vi "Wire All Terminals_core.vi"(8 "error in (no error)":errorcluster, 9 "User string":string, 10 "Create constants?":bool, 11 "SelList[]":refnum<vi>[](array[refnum])) -> (0 "error out":errorcluster, 3 "changes made?":bool)   [LabVIEW 2017]
doc: "Creates controls and indicators for all unwired inputs and outputs of the selected block diagram object(s). If 'shift' is also pressed, creates constants for all unwired inputs of the selected block diagram object(s).\n\nDefault Shortcut - [D]"
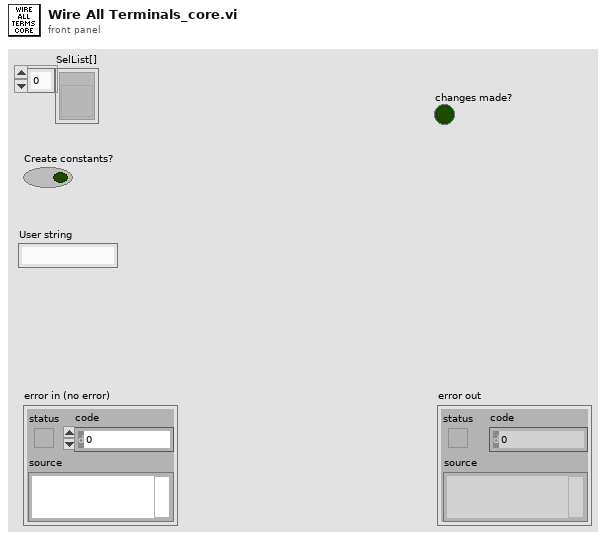
[diagram p1: front panel]
types:
  T1 = enum16{"Invalid Wire Rule", "Required", "Recommended", "Optional", "Dynamic Dispatch"}[]
  T2 = typedef "VariantType.lvlib/Type.ctl" = enum8{"Invalid Type", "Void", "I8", "I16", "I32", "I64", "U8", "U16", "U32", "U64", "Single Float", "Double Float", "Extended Float", "Single Complex", "Double Complex", "Extended Complex", "Enum U8", "Enum U16", "Enum U32", "Enum U64", "Single Float With Unit", "Double Float With Unit", "Extended Float With Unit", "Single Complex with Unit", "Double Complex with Unit", "Extended Complex with Unit", "Boolean", "String", "Path", "Picture", "Tag", "Array", "Cluster", "Variant", "LV Variant", "Waveform", "Timestamp", "Digital Waveform", "Digital Data", "ExpressData", "Refnum", "External Data", "VI", "Poly VI", "LabVIEW Class Instance", "Fixed Point"}
  T3 = enum16{"Invalid Wire Rule", "Required", "Recommended", "Optional"}
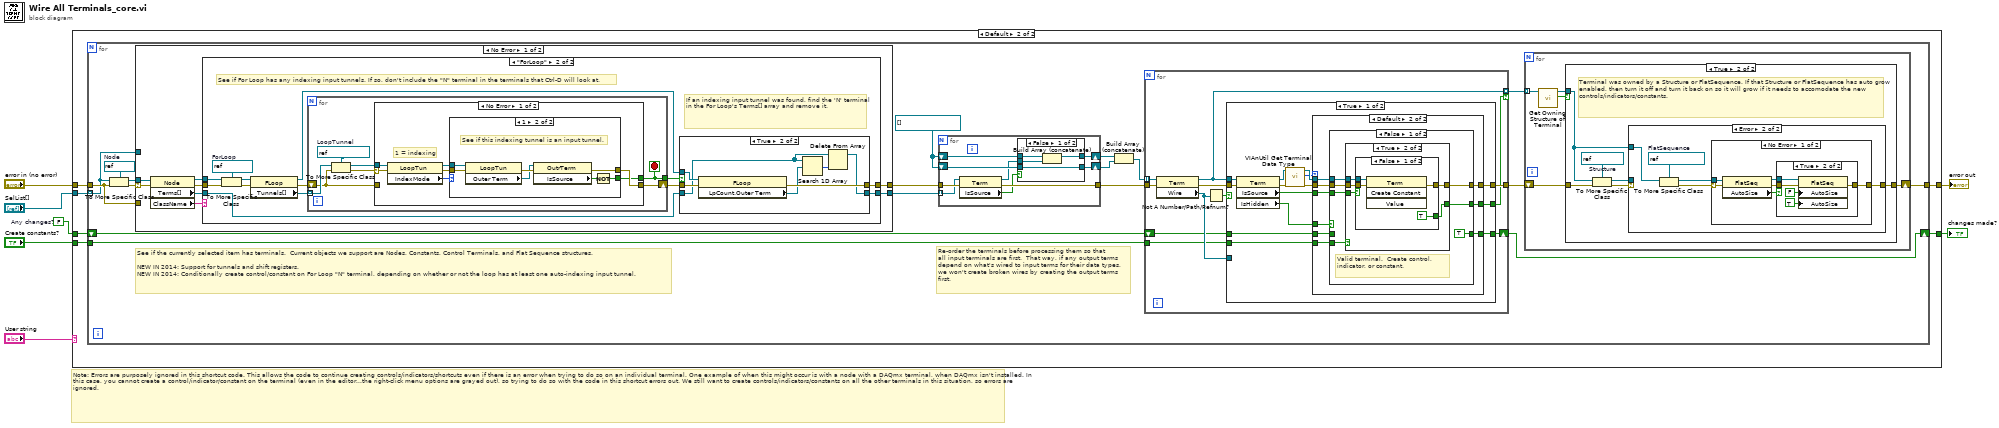
[diagram p0: block diagram]
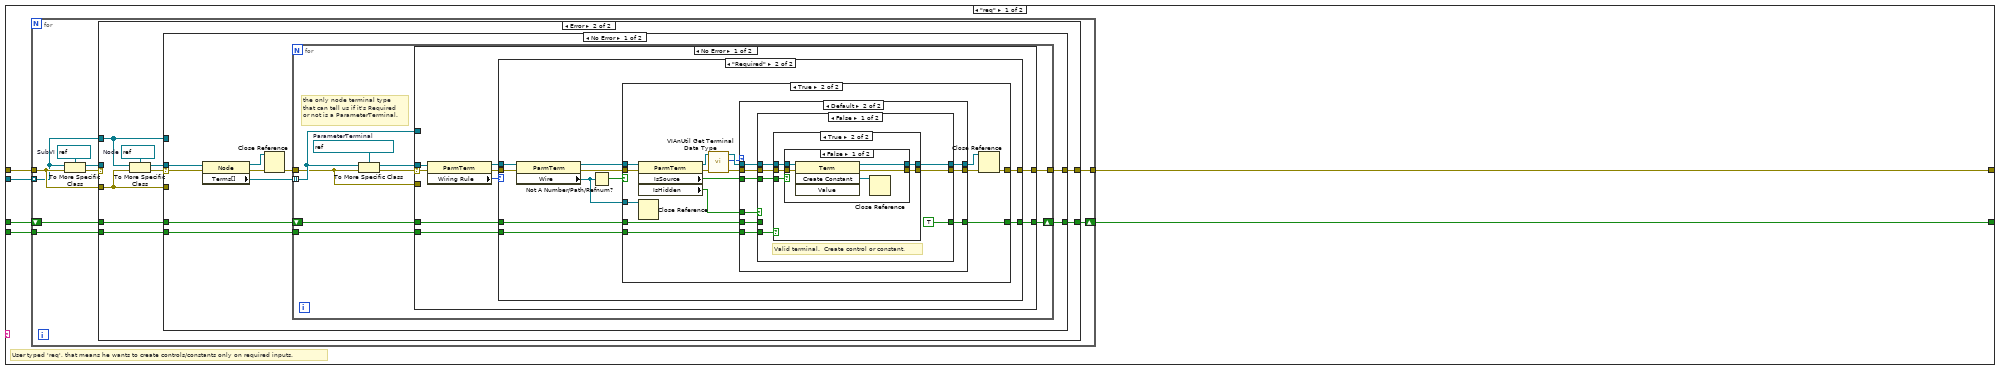
[diagram p2: hidden frame]
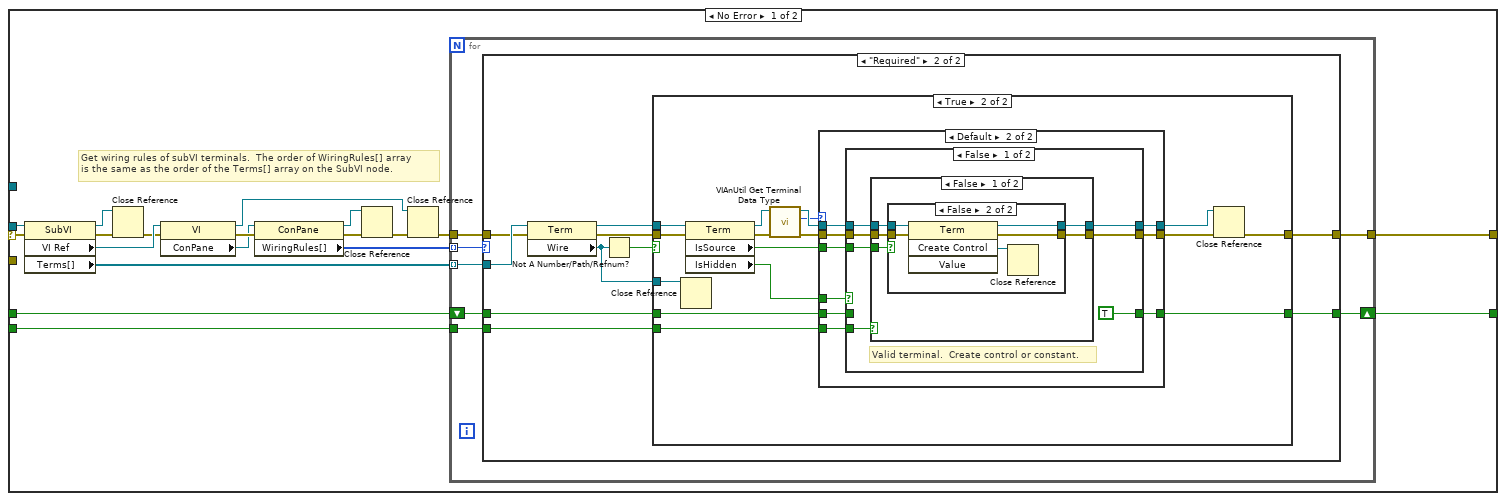
[diagram p3: hidden frame]
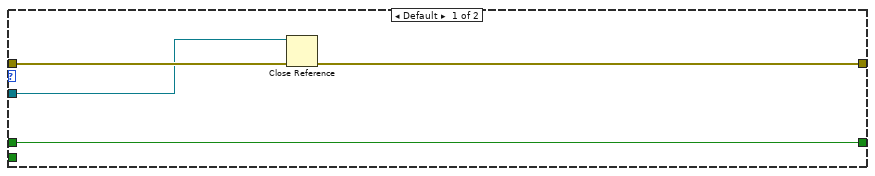
[diagram p4: hidden frame]
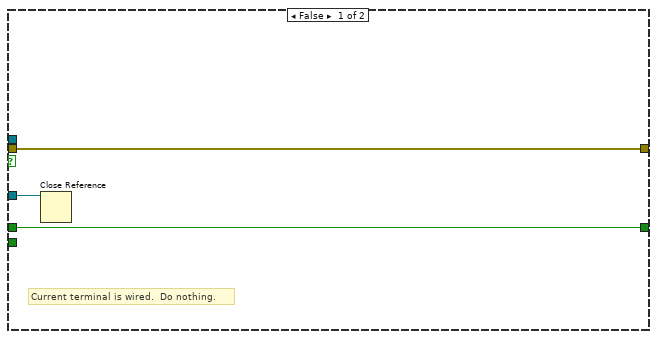
[diagram p5: hidden frame]
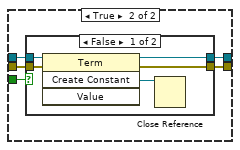
[diagram p8: hidden frame]
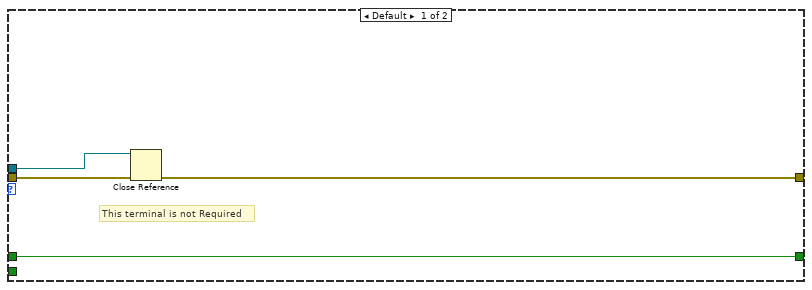
[diagram p11: hidden frame]
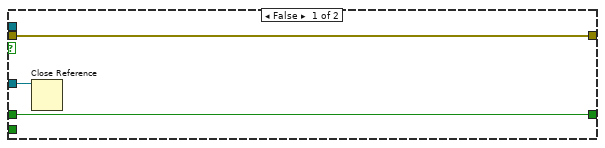
[diagram p12: hidden frame]
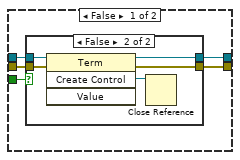
[diagram p14: hidden frame]
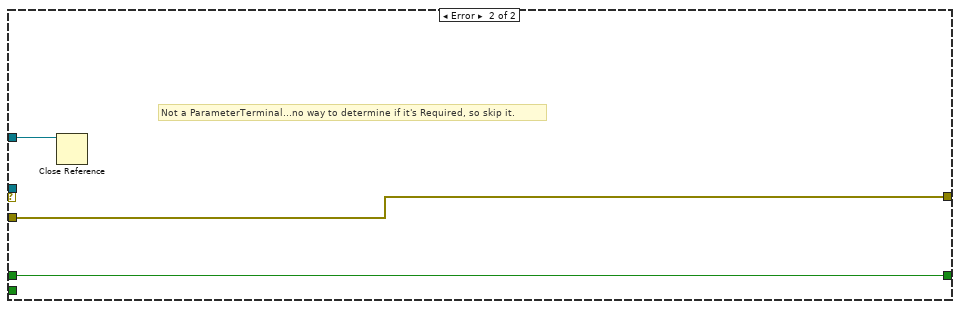
[diagram p18: hidden frame]
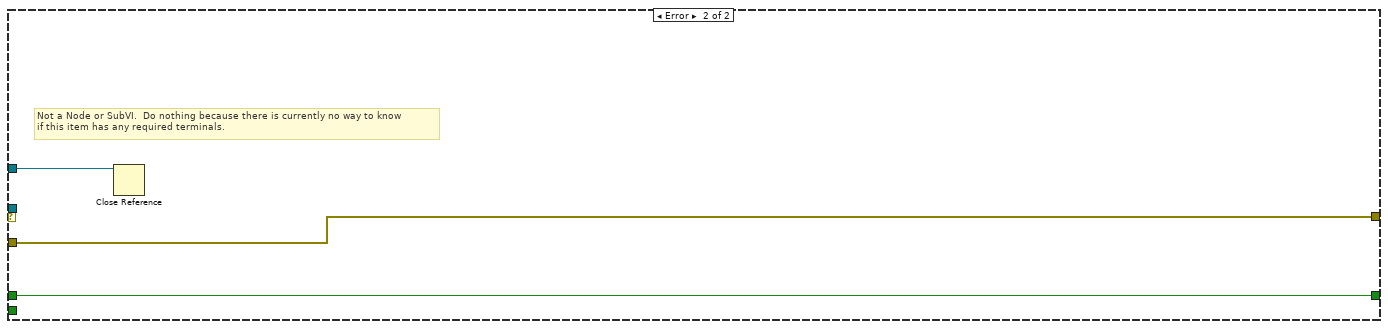
[diagram p19: hidden frame]
diagram:
  w7 = FALSE  # Any changes?
  # "Note: Errors are purposely ignored in this shortcut code. This allows the code to continue creating controls/indicators/shortcuts even if there is an error when trying to do so on an individual terminal. One example of when this might occur is with a node with a DAQmx terminal, when DAQmx isn't installed. In this case, you cannot create a control/indicator/constant on the terminal (even in the editor...the right-click menu options are grayed out), so trying to do so with the code in this shortcut errors out. We still want to create controls/indicators/constants on all the other terminals in this situation, so errors are ignored."
  n1 = case shown="Default" "User string" {
    tunnel: "Create constants?" -> [w8 w255]
    tunnel: w7 -> [w13 w254]
    tunnel: [w12 w253] -> w4
    tunnel: [w9 w252] -> w5
    tunnel: "SelList[]" -> [w11 w251]
    tunnel: "error in (no error)" -> [w10 w250]
    frame "req" {
      # "User typed 'req', that means he wants to create controls/constants only on required inputs."
      n2 = for {
        shift-right: [w17] -> w12
        shift-left: w13 -> [w19]
        tunnel: w11 -> [w14] mode=indexing
        tunnel: w8 -> [w16]
        tunnel: w10 -> [w15]
        tunnel: [w18] -> w9
        w22 = refnum<vi> refnum  # SubVI
        n3 = To More Specific Class(target class=w22, reference=w14, error in=w15) -> (specific class reference=w20:refnum<vi>, error out=w21:errorcluster)
        n4 = case shown="Error" w21 {
          selector: w21 -> [w40 _]
          tunnel: w20 -> [w41 _]
          tunnel: w19 -> [w27 w129]
          tunnel: [w30 w131] -> w18
          tunnel: [w26 w130] -> w17
          tunnel: w16 -> [w25 w128]
          tunnel: w15 -> [_ w134]
          tunnel: w14 -> [_ w132]
          frame No Error {
            # "Get wiring rules of subVI terminals.  The order of WiringRules[] array\nis the same as the order of the Terms[] array on the SubVI node."
            n5 = property class="SubVI"(reference=w41, error in=w40) -> (reference out=w23:refnum<vi>, error out=w39:errorcluster, "VI Ref"=w38:refnum<vi>, "Terms[]"=w28:refnum<vi>[])
            n6 = Close Reference(reference=w23, error in (no error)=w39) -> (error out=w24:errorcluster)
            n7 = property class="VI"(reference=w38, error in=w24) -> (reference out=w32:refnum<vi>, error out=w37:errorcluster, "ConPane"=w36:refnum<vi>)
            n8 = property class="ConPane"(reference=w36, error in=w37) -> (reference out=w34:refnum<vi>, error out=w35:errorcluster, "WiringRules[]"=w29:T1)
            n9 = Close Reference(reference=w34, error in (no error)=w35) -> (error out=w33:errorcluster)
            n10 = Close Reference(reference=w32, error in (no error)=w33) -> (error out=w31:errorcluster)
            n11 = for {
              tunnel: w29 -> [w47] mode=indexing
              tunnel: w28 -> [w46] mode=indexing
              shift-right: [w43] -> w26
              shift-left: w27 -> [w44]
              tunnel: w25 -> [w42]
              tunnel: w31 -> [w48]
              tunnel: [w45] -> w30
              n12 = case shown="\"Required\"" w47 {
                tunnel: w48 -> [w52 w54]
                tunnel: w46 -> [w49 w58]
                tunnel: [w51 w59] -> w45
                tunnel: w44 -> [w50 w62]
                tunnel: [w50 w60] -> w43
                tunnel: w42 -> [_ w61]
                frame Default {
                  n13 = Close Reference(reference=w49, error in (no error)=w52) -> (error out=w51:errorcluster)
                }
                frame "Required" {
                  n14 = property class="Term"(reference=w58, error in=w54) -> (reference out=w57:refnum<vi>, error out=w53:errorcluster, "Wire"=w55:refnum<vi>)
                  n15 = Not A Number/Path/Refnum?(number/path/refnum=w55) -> (NaN/Path/Refnum?=w56:bool)
                  n16 = case shown="True" w56 {
                    tunnel: w62 -> [w63 w77]
                    tunnel: w61 -> [_ w76]
                    tunnel: [w63 w75] -> w60
                    tunnel: [w64 w74] -> w59
                    tunnel: w53 -> [w64 w73]
                    tunnel: w57 -> [_ w67]
                    tunnel: w55 -> [w65 w66]
                    frame False {
                      # "Current terminal is wired.  Do nothing."
                      n17 = Close Reference(reference=w65) -> ()  [unwired: 1 in, 1 out]
                    }
                    frame True {
                      n18 = Close Reference(reference=w66) -> ()  [unwired: 1 in, 1 out]
                      n19 = property class="Term"(reference=w67, error in=w73) -> (reference out=w70:refnum<vi>, error out=w72:errorcluster, "IsSource"=w81:bool, "IsHidden"=w78:bool)
                      n20 = call <vilib>:"VIAnUtil Get Terminal Data Type.vi"("error in (no error)"=w72, "Terminal"=w70) -> ("error out"=w71:errorcluster, "Data Type"=w68:T2, "dup  Terminal"=w69:refnum<vi>)  [unwired: 6 in, 1 out]
                      n21 = case shown="Default" w68 {
                        tunnel: [w84 w93] -> w75
                        tunnel: w81 -> [_ w92]
                        tunnel: w69 -> [w82 w91]
                        tunnel: [w83 w90] -> w80
                        tunnel: [w82 w89] -> w79
                        tunnel: w71 -> [w83 w88]
                        tunnel: w77 -> [w84 w85]
                        tunnel: w76 -> [_ w87]
                        tunnel: w78 -> [_ w86]
                        frame "Invalid Type", "Void" {
                          # "Current terminal is void (like an empty terminal on\na subVI).  Do nothing."
                        }
                        frame Default {
                          n22 = case shown="False" w86 {
                            tunnel: [TRUE w125] -> w93
                            tunnel: w92 -> [w99 _]
                            tunnel: w91 -> [w98 w126]
                            tunnel: [w97 w127] -> w90
                            tunnel: [w96 w126] -> w89
                            tunnel: w88 -> [w95 w127]
                            tunnel: w87 -> [w94 _]
                            tunnel: w85 -> [_ w125]
                            frame False {
                              # "Valid terminal.  Create control or constant."
                              n23 = case shown="False" w94 {
                                tunnel: w99 -> [w105 w117]
                                tunnel: w98 -> [w104 w116]
                                tunnel: [w103 w115] -> w97
                                tunnel: [w102 w114] -> w96
                                tunnel: w95 -> [w101 w113]
                                frame False {
                                n24 = case shown="False" w105 {
                                tunnel: w101 -> [w106 w112]
                                tunnel: w104 -> [w107 w110]
                                tunnel: [w106 w111] -> w103
                                tunnel: [w107 w109] -> w102
                                frame True {
                                }
                                frame False {
                                n25 = invoke class="Term" method="Create Control"(reference=w110, error in=w112) -> (reference out=w109:refnum<vi>, error out=w111:errorcluster, "Create Control"=w108:refnum<vi>)  [unwired: 2 in, 1 out]
                                n26 = Close Reference(reference=w108) -> ()  [unwired: 1 in, 1 out]
                                }
                                }
                                }
                                frame True {
                                n27 = case shown="False" w117 {
                                tunnel: w113 -> [w122 w124]
                                tunnel: w116 -> [w120 w123]
                                tunnel: [w121 w124] -> w115
                                tunnel: [w119 w123] -> w114
                                frame False {
                                n28 = invoke class="Term" method="Create Constant"(reference=w120, error in=w122) -> (reference out=w119:refnum<vi>, error out=w121:errorcluster, "Create Constant"=w118:refnum<vi>)  [unwired: 2 in, 1 out]
                                n29 = Close Reference(reference=w118) -> ()  [unwired: 1 in, 1 out]
                                }
                                frame True {
                                }
                                }
                                }
                              }
                            }
                            frame True {
                              # "Do not attempt to create inputs/outputs\non hidden terminals (like Dynamic Event terms\non an Event Structure that aren't showing)"
                            }
                          }
                        }
                      }
                      n30 = Close Reference(reference=w79, error in (no error)=w80) -> (error out=w74:errorcluster)
                    }
                  }
                }
              }
            }
          }
          frame Error {
            w136 = refnum<vi> refnum  # Node
            n31 = To More Specific Class(target class=w136, reference=w132, error in=w134) -> (specific class reference=w133:refnum<vi>, error out=w135:errorcluster)
            n32 = case shown="No Error" w135 {
              selector: w135 -> [w146 _]
              tunnel: w134 -> [_ w248]
              tunnel: w133 -> [w145 _]
              tunnel: w132 -> [_ w249]
              tunnel: [w138 w248] -> w131
              tunnel: [w139 w247] -> w130
              tunnel: w129 -> [w140 w247]
              tunnel: w128 -> [w137 _]
              frame No Error {
                n33 = property class="Node"(reference=w145, error in=w146) -> (reference out=w143:refnum<vi>, error out=w144:errorcluster, "Terms[]"=w141:refnum<vi>[])
                n34 = Close Reference(reference=w143, error in (no error)=w144) -> (error out=w142:errorcluster)
                n35 = for {
                  tunnel: w141 -> [w150] mode=indexing
                  shift-right: [w151] -> w139
                  shift-left: w140 -> [w152]
                  tunnel: w137 -> [w147]
                  tunnel: w142 -> [w149]
                  tunnel: [w148] -> w138
                  w155 = refnum<vi> refnum  # ParameterTerminal
                  # "the only node terminal type\nthat can tell us if it's Required\nor not is a ParameterTerminal."
                  n36 = To More Specific Class(target class=w155, reference=w150, error in=w149) -> (specific class reference=w153:refnum<vi>, error out=w154:errorcluster)
                  n37 = case shown="No Error" w154 {
                    selector: w154 -> [w164 _]
                    tunnel: w153 -> [w163 _]
                    tunnel: w152 -> [w162 w246]
                    tunnel: [w157 w246] -> w151
                    tunnel: w150 -> [_ w245]
                    tunnel: w149 -> [_ w244]
                    tunnel: [w158 w244] -> w148
                    tunnel: w147 -> [w156 _]
                    frame No Error {
                      n38 = property class="ParmTerm"(reference=w163, error in=w164) -> (reference out=w159:refnum<vi>, error out=w160:errorcluster, "Wiring Rule"=w161:T3)
                      n39 = case shown="\"Required\"" w161 {
                        tunnel: w162 -> [w165 w178]
                        tunnel: w160 -> [w168 w172]
                        tunnel: w159 -> [w167 w174]
                        tunnel: [w166 w176] -> w158
                        tunnel: [w165 w177] -> w157
                        tunnel: w156 -> [_ w175]
                        frame Default {
                          # "This terminal is not Required"
                          n40 = Close Reference(reference=w167, error in (no error)=w168) -> (error out=w166:errorcluster)
                        }
                        frame "Required" {
                          n41 = property class="ParmTerm"(reference=w174, error in=w172) -> (reference out=w173:refnum<vi>, error out=w171:errorcluster, "Wire"=w169:refnum<vi>)
                          n42 = Not A Number/Path/Refnum?(number/path/refnum=w169) -> (NaN/Path/Refnum?=w170:bool)
                          n43 = case shown="True" w170 {
                            tunnel: w173 -> [_ w193]
                            tunnel: w178 -> [w181 w192]
                            tunnel: [w181 w191] -> w177
                            tunnel: [w180 w190] -> w176
                            tunnel: w175 -> [_ w189]
                            tunnel: w171 -> [w180 w188]
                            tunnel: w169 -> [w179 w182]
                            frame False {
                              n44 = Close Reference(reference=w179) -> ()  [unwired: 1 in, 1 out]
                            }
                            frame True {
                              n45 = property class="ParmTerm"(reference=w193, error in=w188) -> (reference out=w186:refnum<vi>, error out=w187:errorcluster, "IsSource"=w197:bool, "IsHidden"=w194:bool)
                              n46 = Close Reference(reference=w182) -> ()  [unwired: 1 in, 1 out]
                              n47 = call <vilib>:"VIAnUtil Get Terminal Data Type.vi"("error in (no error)"=w187, "Terminal"=w186) -> ("error out"=w184:errorcluster, "Data Type"=w183:T2, "dup  Terminal"=w185:refnum<vi>)  [unwired: 6 in, 1 out]
                              n48 = case shown="Default" w183 {
                                tunnel: [w200 w209] -> w191
                                tunnel: w197 -> [_ w208]
                                tunnel: w185 -> [w198 w207]
                                tunnel: [w199 w206] -> w196
                                tunnel: [w198 w205] -> w195
                                tunnel: w184 -> [w199 w204]
                                tunnel: w192 -> [w200 w201]
                                tunnel: w189 -> [_ w203]
                                tunnel: w194 -> [_ w202]
                                frame "Invalid Type", "Void" {
                                # "Current terminal is void (like an empty terminal on\na subVI).  Do nothing."
                                }
                                frame Default {
                                n49 = case shown="False" w202 {
                                tunnel: [TRUE w241] -> w209
                                tunnel: w208 -> [w215 _]
                                tunnel: w207 -> [w214 w242]
                                tunnel: [w213 w243] -> w206
                                tunnel: [w212 w242] -> w205
                                tunnel: w204 -> [w211 w243]
                                tunnel: w203 -> [w210 _]
                                tunnel: w201 -> [_ w241]
                                frame False {
                                # "Valid terminal.  Create control or constant."
                                n50 = case shown="True" w210 {
                                tunnel: w215 -> [w221 w233]
                                tunnel: w214 -> [w220 w232]
                                tunnel: [w219 w231] -> w213
                                tunnel: [w218 w230] -> w212
                                tunnel: w211 -> [w217 w229]
                                frame False {
                                n51 = case shown="False" w221 {
                                tunnel: w217 -> [w222 w228]
                                tunnel: w220 -> [w223 w226]
                                tunnel: [w222 w227] -> w219
                                tunnel: [w223 w225] -> w218
                                frame True {
                                }
                                frame False {
                                n52 = invoke class="Term" method="Create Control"(reference=w226, error in=w228) -> (reference out=w225:refnum<vi>, error out=w227:errorcluster, "Create Control"=w224:refnum<vi>)  [unwired: 2 in, 1 out]
                                n53 = Close Reference(reference=w224) -> ()  [unwired: 1 in, 1 out]
                                }
                                }
                                }
                                frame True {
                                n54 = case shown="False" w233 {
                                tunnel: w229 -> [w238 w240]
                                tunnel: w232 -> [w236 w239]
                                tunnel: [w237 w240] -> w231
                                tunnel: [w235 w239] -> w230
                                frame False {
                                n55 = invoke class="Term" method="Create Constant"(reference=w236, error in=w238) -> (reference out=w235:refnum<vi>, error out=w237:errorcluster, "Create Constant"=w234:refnum<vi>)  [unwired: 2 in, 1 out]
                                n56 = Close Reference(reference=w234) -> ()  [unwired: 1 in, 1 out]
                                }
                                frame True {
                                }
                                }
                                }
                                }
                                }
                                frame True {
                                # "Do not attempt to create inputs/outputs\non hidden terminals (like Dynamic Event terms\non an Event Structure that aren't showing)"
                                }
                                }
                                }
                              }
                              n57 = Close Reference(reference=w195, error in (no error)=w196) -> (error out=w190:errorcluster)
                            }
                          }
                        }
                      }
                    }
                    frame Error {
                      # "Not a ParameterTerminal...no way to determine if it's Required, so skip it."
                      n58 = Close Reference(reference=w245) -> ()  [unwired: 1 in, 1 out]
                    }
                  }
                }
              }
              frame Error {
                # "Not a Node or SubVI.  Do nothing because there is currently no way to know\nif this item has any required terminals."
                n59 = Close Reference(reference=w249) -> ()  [unwired: 1 in, 1 out]
              }
            }
          }
        }
      }
    }
    frame Default {
      n60 = for {
        tunnel: w251 -> [w267] mode=indexing
        shift-right: [w256] -> w253
        shift-left: w254 -> [w271]
        tunnel: w255 -> [w270]
        tunnel: w250 -> [w269]
        tunnel: [w258] -> w252
        w262 = refnum<vi>[] [] ("Terms[]")
        w273 = refnum<vi> refnum  # Node
        # "Re-order the terminals before processing them so that\nall input terminals are first.  That way, if any output terms\ndepend on what's wired to input terms for their data types,\nwe won't create broken wires by creating the output terms\nfirst."
        # "See if the currently selected item has terminals.  Current objects we support are Nodes, Constants, Control Terminals, and Flat Sequence structures.\n\nNEW IN 2014: Support for tunnels and shift registers.\nNEW IN 2014: Conditionally create control/constant on For Loop \"N\" terminal, depending on whether or not the loop has at least one auto-indexing input tunnel."
        n61 = To More Specific Class(target class=w273, reference=w267, error in=w269) -> (specific class reference=w272:refnum<vi>, error out=w268:errorcluster)
        n62 = case shown="No Error" w268 {
          selector: w268 -> [w338 _]
          tunnel: w272 -> [w339 _]
          tunnel: [w333 w388] -> w265
          tunnel: [w334 w389] -> w266
          tunnel: w269 -> [_ w390]
          tunnel: w267 -> [_ w387]
          frame No Error {
            n63 = property class="Node"(reference=w339, error in=w338) -> (reference out=w332:refnum<vi>, error out=w335:errorcluster, "Terms[]"=w336:refnum<vi>[], "ClassName"=w337:string)
            n64 = case shown="\"ForLoop\"" w337 {
              tunnel: w336 -> [w340 w345]
              tunnel: w335 -> [w341 w354]
              tunnel: [w341 w343] -> w334
              tunnel: [w340 w344] -> w333
              tunnel: w332 -> [_ w353]
              frame Default {
                # "Node is not a For Loop."
              }
              frame "ForLoop" {
                w352 = refnum<vi> refnum  # ForLoop
                # "If an indexing input tunnel was found, find the 'N' terminal in the For Loop's Terms[] array and remove it."
                # "See if For Loop has any indexing input tunnels. If so, don't include the \"N\" terminal in the terminals that Ctrl-D will look at."
                n65 = To More Specific Class(target class=w352, reference=w353, error in=w354) -> (specific class reference=w350:refnum<vi>, error out=w351:errorcluster)
                n66 = property class="FLoop"(reference=w350, error in=w351) -> (reference out=w342:refnum<vi>, error out=w349:errorcluster, "Tunnels[]"=w348:refnum<vi>[])
                n67 = for {
                  shift-right: [w365] -> w347
                  shift-left: w349 -> [w368]
                  tunnel: w348 -> [w369] mode=indexing
                  tunnel: [w364] -> w346
                  stop <- w364 stop-if-true
                  w370 = refnum<vi> refnum  # LoopTunnel
                  n68 = To More Specific Class(target class=w370, reference=w369, error in=w368) -> (specific class reference=w366:refnum<vi>, error out=w367:errorcluster)
                  n69 = case shown="No Error" w367 {
                    selector: w367 -> [w377 _]
                    tunnel: w368 -> [_ w386]
                    tunnel: w366 -> [w376 _]
                    tunnel: [w372 w386] -> w365
                    tunnel: [w371 _] -> w364
                    frame No Error {
                      # "1 = indexing"
                      n70 = property class="LoopTun"(reference=w376, error in=w377) -> (reference out=w373:refnum<vi>, error out=w374:errorcluster, "IndexMode"=w375:u32)
                      n71 = case shown="1" w375 {
                        tunnel: w374 -> [w378 w385]
                        tunnel: w373 -> [_ w384]
                        tunnel: [w378 w381] -> w372
                        tunnel: [_ w379] -> w371
                        frame Default {
                          # "Not an indexing loop tunnel"
                        }
                        frame 1 {
                          # "See if this indexing tunnel is an input tunnel."
                          n72 = property class="LoopTun"(reference=w384, error in=w385) -> (error out=w383:errorcluster, "Outer Term"=w382:refnum<vi>)  [unwired: 1 out]
                          n73 = property class="OutrTerm"(reference=w382, error in=w383) -> (error out=w381:errorcluster, "IsSource"=w380:bool)  [unwired: 1 out]
                          n74 = Not(x=w380) -> (.not. x?=w379:bool)
                        }
                      }
                    }
                    frame Error {
                      # "Not a LoopTunnel, so indexing can't be set on it."
                    }
                  }
                }
                n75 = case shown="True" w346 {
                  tunnel: w347 -> [w355 w363]
                  tunnel: w345 -> [w356 w358]
                  tunnel: [w356 w357] -> w344
                  tunnel: [w355 w361] -> w343
                  tunnel: w342 -> [_ w362]
                  frame False {
                  }
                  frame True {
                    n76 = property class="FLoop"(reference=w362, error in=w363) -> (error out=w361:errorcluster, "LpCount.Outer Term"=w360:refnum<vi>)  [unwired: 1 out]
                    n77 = Search 1D Array(1D array=w358, element=w360) -> (index of element=w359:i32)  [unwired: 1 in]
                    n78 = Delete From Array(array=w358, index=w359) -> (array with subset deleted=w357:refnum<vi>[])  [unwired: 1 in, 1 out]
                  }
                }
              }
            }
          }
          frame Error {
            w393 = refnum<vi> refnum  # Constant
            n79 = To More Specific Class(target class=w393, reference=w387, error in=w390) -> (specific class reference=w391:refnum<vi>, error out=w392:errorcluster)
            n80 = case shown="Error" w392 {
              selector: w392 -> [w400 _]
              tunnel: w390 -> [_ w402]
              tunnel: w391 -> [w399 _]
              tunnel: [w394 w404] -> w389
              tunnel: [w397 w403] -> w388
              tunnel: w387 -> [_ w401]
              frame No Error {
                n81 = property class="Const"(reference=w399, error in=w400) -> (reference out=w395:refnum<vi>, error out=w396:errorcluster, "Terminal"=w398:refnum<vi>)
                n82 = Close Reference(reference=w395, error in (no error)=w396) -> (error out=w394:errorcluster)
                n83 = Build Array(w398) -> (w397:refnum<vi>[])
              }
              frame Error {
                w407 = refnum<vi> refnum  # Terminal
                n84 = To More Specific Class(target class=w407, reference=w401, error in=w402) -> (specific class reference=w405:refnum<vi>, error out=w406:errorcluster)
                n85 = case shown="Error" w406 {
                  selector: w406 -> [w410 _]
                  tunnel: w405 -> [w409 _]
                  tunnel: [w410 w413] -> w404
                  tunnel: [w408 w412] -> w403
                  tunnel: w402 -> [_ w414]
                  tunnel: w401 -> [_ w411]
                  frame No Error {
                    n86 = Build Array(w409) -> (w408:refnum<vi>[])
                  }
                  frame Error {
                    w417 = refnum<vi> refnum  # FlatSequence
                    n87 = To More Specific Class(target class=w417, reference=w411, error in=w414) -> (specific class reference=w415:refnum<vi>, error out=w416:errorcluster)
                    n88 = case shown="Error" w416 {
                      selector: w416 -> [w423 _]
                      tunnel: w415 -> [w422 _]
                      tunnel: w414 -> [_ w426]
                      tunnel: [w418 w425] -> w413
                      tunnel: [w421 w424] -> w412
                      tunnel: w411 -> [_ w427]
                      frame No Error {
                        n89 = property class="FlatSeq"(reference=w422, error in=w423) -> (reference out=w419:refnum<vi>, error out=w420:errorcluster, "Terms[]"=w421:refnum<vi>[])
                        n90 = Close Reference(reference=w419, error in (no error)=w420) -> (error out=w418:errorcluster)
                      }
                      frame Error {
                        w430 = refnum<vi> refnum  # Tunnel
                        n91 = To More Specific Class(target class=w430, reference=w427, error in=w426) -> (specific class reference=w428:refnum<vi>, error out=w429:errorcluster)
                        n92 = case shown="No Error" w429 {
                          selector: w429 -> [w435 _]
                          tunnel: w428 -> [w434 _]
                          tunnel: w427 -> [_ _]
                          tunnel: w426 -> [_ w436]
                          tunnel: [w433 w436] -> w425
                          tunnel: [w431 _] -> w424
                          frame No Error {
                            # "Get the outside terminal of any selected tunnel. This also includes shift registers (they inherit from the Tunnel class)."
                            n93 = property class="Tun"(reference=w434, error in=w435) -> (error out=w433:errorcluster, "Outer Term"=w432:refnum<vi>)  [unwired: 1 out]
                            n94 = Build Array(w432) -> (w431:refnum<vi>[])
                          }
                          frame Error {
                            # "Not a supported type for this shortcut."
                          }
                        }
                      }
                    }
                  }
                }
              }
            }
          }
        }
        n95 = for {
          tunnel: w265 -> [w322] mode=indexing
          shift-right: [w318] -> w261
          shift-left: w262 -> [w320]
          shift-right: [w317] -> w260
          shift-left: w262 -> [w319]
          tunnel: w266 -> [w323]
          tunnel: [w321] -> w264
          n96 = property class="Term"(reference=w322, error in=w323) -> (reference out=w316:refnum<vi>, error out=w321:errorcluster, "IsSource"=w315:bool)
          n97 = case shown="False" w315 {
            tunnel: w320 -> [w327 w331]
            tunnel: w319 -> [w325 w330]
            tunnel: [w326 w331] -> w318
            tunnel: [w325 w329] -> w317
            tunnel: w316 -> [w324 w328]
            frame False {
              n98 = Build Array (concatenate)(w327, w324) -> (w326:refnum<vi>[])
            }
            frame True {
              n99 = Build Array (concatenate)(w330, w328) -> (w329:refnum<vi>[])
            }
          }
        }
        n100 = Build Array (concatenate)(w261, w260) -> (w263:refnum<vi>[])
        n101 = for {
          tunnel: w263 -> [w446] mode=indexing
          shift-right: [w441] -> w256
          shift-left: w271 -> [w442]
          tunnel: w270 -> [w439]
          tunnel: w264 -> [w447]
          tunnel: [w440] -> w259
          tunnel: [w438] -> w257 mode=indexing if=w437
          n102 = property class="Term"(reference=w446, error in=w447) -> (reference out=w438:refnum<vi>, error out=w445:errorcluster, "Wire"=w443:refnum<vi>)
          n103 = Not A Number/Path/Refnum?(number/path/refnum=w443) -> (NaN/Path/Refnum?=w444:bool)
          n104 = case shown="True" w444 {
            tunnel: w445 -> [w461 w505]
            tunnel: w438 -> [w460 _]
            tunnel: w443 -> [_ _]
            tunnel: w442 -> [w457 w506]
            tunnel: [w459 w506] -> w441
            tunnel: [w449 w505] -> w440
            tunnel: w439 -> [w456 _]
            tunnel: [w448 _] -> w437
            frame True {
              n105 = property class="Term"(reference=w460, error in=w461) -> (reference out=w452:refnum<vi>, error out=w454:errorcluster, "IsSource"=w458:bool, "IsHidden"=w455:bool)
              n106 = call <vilib>:"VIAnUtil Get Terminal Data Type.vi"("error in (no error)"=w454, "Terminal"=w452) -> ("error out"=w453:errorcluster, "Data Type"=w450:T2, "dup  Terminal"=w451:refnum<vi>)  [unwired: 6 in, 1 out]
              n107 = case shown="Default" w450 {
                tunnel: [w463 w472] -> w459
                tunnel: w458 -> [_ w471]
                tunnel: w451 -> [_ w470]
                tunnel: [w462 w469] -> w449
                tunnel: w453 -> [w462 w468]
                tunnel: w457 -> [w463 w465]
                tunnel: w456 -> [_ w467]
                tunnel: w455 -> [_ w466]
                tunnel: [_ w464] -> w448
                frame "Invalid Type", "Void" {
                  # "Current terminal is void (like an empty terminal on a subVI).  Do nothing."
                }
                frame Default {
                  n108 = case shown="False" w466 {
                    tunnel: [TRUE w503] -> w472
                    tunnel: w471 -> [w478 _]
                    tunnel: w470 -> [w477 _]
                    tunnel: [w476 w504] -> w469
                    tunnel: w468 -> [w475 w504]
                    tunnel: w467 -> [w474 _]
                    tunnel: w465 -> [_ w503]
                    tunnel: [w473 _] -> w464
                    frame False {
                      # "Valid terminal.  Create control, indicator, or constant."
                      n109 = case shown="True" w474 {
                        tunnel: w478 -> [w484 w497]
                        tunnel: w477 -> [w483 w496]
                        tunnel: [w482 w495] -> w476
                        tunnel: w475 -> [w481 w494]
                        tunnel: [TRUE w493] -> w473
                        frame False {
                          n110 = case shown="False" w484 {
                            tunnel: w481 -> [w488 w492]
                            tunnel: w483 -> [w486 w490]
                            tunnel: [w487 w491] -> w482
                            tunnel: [w485 w489] -> _
                            frame True {
                              n111 = invoke class="Term" method="Create Indicator"(reference=w486, error in=w488) -> (reference out=w485:refnum<vi>, error out=w487:errorcluster)  [unwired: 1 in, 1 out]
                            }
                            frame False {
                              n112 = invoke class="Term" method="Create Control"(reference=w490, error in=w492) -> (reference out=w489:refnum<vi>, error out=w491:errorcluster)  [unwired: 2 in, 2 out]
                            }
                          }
                        }
                        frame True {
                          n113 = case shown="False" w497 {
                            tunnel: w494 -> [w501 w502]
                            tunnel: w496 -> [w499 _]
                            tunnel: [w500 w502] -> w495
                            tunnel: [TRUE _] -> w493
                            frame False {
                              n114 = invoke class="Term" method="Create Constant"(reference=w499, error in=w501) -> (error out=w500:errorcluster)  [unwired: 2 in, 3 out]
                            }
                            frame True {
                            }
                          }
                        }
                      }
                    }
                    frame True {
                      # "Do not attempt to create inputs/outputs on hidden terminals (like Dynamic Event terms on an Event Structure that aren't showing)"
                    }
                  }
                }
              }
            }
            frame False {
              # "Current terminal is wired.  Do nothing."
            }
          }
        }
        n115 = for {
          shift-right: [w274] -> w258
          shift-left: w259 -> [w275]
          tunnel: w257 -> [w278] mode=indexing
          n116 = call <vilib>:"Get Owning Structure of Terminal.vi"("Terminal"=w278) -> ("Terminal Owned by Structure?"=w277:bool, "Owning Structure"=w276:refnum<vi>)  [unwired: 9 in]
          n117 = case shown="True" w277 {
            tunnel: w276 -> [_ w280]
            tunnel: w275 -> [w279 w285]
            tunnel: [w279 w281] -> w274
            frame False {
              # "Terminal was not owned at any point in its hierarchy by a Structure or FlatSequence. This terminal must be on the top-level diagram (or its owning Node is on the top-level diagram)."
            }
            frame True {
              w282 = refnum<vi> refnum  # Structure
              # "Terminal was owned by a Structure or FlatSequence. If that Structure or FlatSequence has auto grow enabled, then turn it off and turn it back on so it will grow if it needs to accomodate the new controls/indicators/constants."
              n118 = To More Specific Class(target class=w282, reference=w280, error in=w285) -> (specific class reference=w283:refnum<vi>, error out=w284:errorcluster)
              n119 = case shown="Error" w284 {
                selector: w284 -> [w291 _]
                tunnel: w283 -> [w290 _]
                tunnel: [w287 w298] -> w281
                tunnel: w280 -> [_ w301]
                frame No Error {
                  n120 = property class="Struct"(reference=w290, error in=w291) -> (reference out=w286:refnum<vi>, error out=w288:errorcluster, "AutoSize"=w289:bool)
                  n121 = case shown="True" w289 {
                    tunnel: w288 -> [w292 w296]
                    tunnel: [w292 w295] -> w287
                    tunnel: w286 -> [_ w297]
                    frame False {
                    }
                    frame True {
                      n122 = property class="Struct"(reference=w297, error in=w296, "AutoSize"=FALSE ("AutoSize To Fit Contents?"), "AutoSize"=TRUE ("AutoSize To Fit Contents?")) -> (error out=w295:errorcluster)  [unwired: 1 out]
                    }
                  }
                }
                frame Error {
                  w302 = refnum<vi> refnum  # FlatSequence
                  n123 = To More Specific Class(target class=w302, reference=w301) -> (specific class reference=w299:refnum<vi>, error out=w300:errorcluster)  [unwired: 1 in]
                  n124 = case shown="No Error" w300 {
                    selector: w300 -> [w305 _]
                    tunnel: w299 -> [w304 _]
                    tunnel: [w303 _] -> w298
                    frame No Error {
                      n125 = property class="FlatSeq"(reference=w304, error in=w305) -> (reference out=w306:refnum<vi>, error out=w307:errorcluster, "AutoSize"=w308:bool)
                      n126 = case shown="True" w308 {
                        tunnel: w307 -> [w309 w313]
                        tunnel: [w309 w312] -> w303
                        tunnel: w306 -> [_ w314]
                        frame False {
                        }
                        frame True {
                          n127 = property class="FlatSeq"(reference=w314, error in=w313, "AutoSize"=FALSE ("AutoSize To Fit Contents?"), "AutoSize"=TRUE ("AutoSize To Fit Contents?")) -> (error out=w312:errorcluster)  [unwired: 1 out]
                        }
                      }
                    }
                    frame Error {
                    }
                  }
                }
              }
            }
          }
        }
      }
    }
  }
  "error out" <- w5
  "changes made?" <- w4
